vi "Select Table.vi"(8 "error in (no error)":errorcluster caption="错误输入（无错误）", 11 "表格":refnum<vi>) -> (0 "error out":errorcluster caption="错误输出")   [LabVIEW 2016]
uses:
  <vilib>/Utility/miscctls.llb/LVRowAndColumnTypeDef.ctl
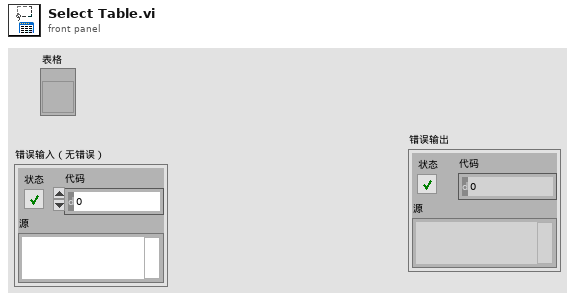
[diagram p1: front panel]
types:
  T1 = typedef "LVRowAndColumnTypeDef.ctl" = cluster{"Row":i32, "Column":i32}
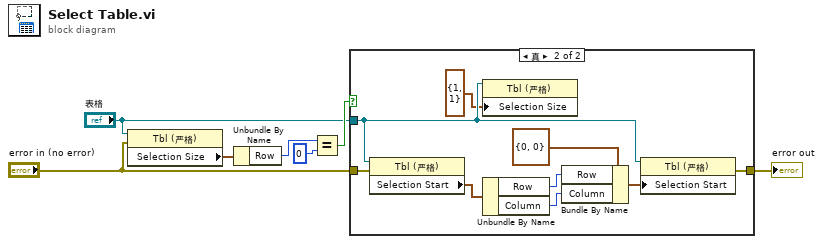
[diagram p0: block diagram]
diagram:
  n1 = property class="Tbl (严格)"(reference="表格", error in="error in (no error)") -> ("Selection Size"=w6:T1)  [unwired: 2 out]
  n2 = Unbundle By Name(w6) -> ("Row"=w5:i32)
  n3 = Equal?(x=w5, y=0) -> (x = y?=w3:bool)
  n4 = case shown="真" w3 {
    tunnel: "error in (no error)" -> [w8 w17]
    tunnel: "表格" -> [_ w11]
    tunnel: [w8 w9] -> w2
    frame False {
    }
    frame True {
      n5 = property class="Tbl (严格)"(reference=w11, error in=w17) -> ("Selection Start"=w16:T1)  [unwired: 2 out]
      n6 = property class="Tbl (严格)"(reference=w11, "Selection Size"=T1 {"Row"=1, "Column"=1} ("选择区域大小")) -> ()  [unwired: 1 in, 2 out]
      n7 = Unbundle By Name(w16) -> ("Row"=w14:i32, "Column"=w13:i32)
      n8 = Bundle By Name(cluster=T1 {"Row"=0, "Column"=0} ("选择区域大小"), "Row"=w14, "Column"=w13) -> (w12:T1)
      n9 = property class="Tbl (严格)"(reference=w11, "Selection Start"=w12) -> (error out=w9:errorcluster)  [unwired: 1 in, 1 out]
    }
  }
  "error out" <- w2
